vi "显示数据写入.vi"(0 "数组":u8[](array[numeric]), 5 "表格控件":string[][](table)) -> (4 "原始值1":string, 6 "实际值1":string, 8 "Function":string, 10 "address":string, 15 "所在表格行数":u16)   [LabVIEW 2018]
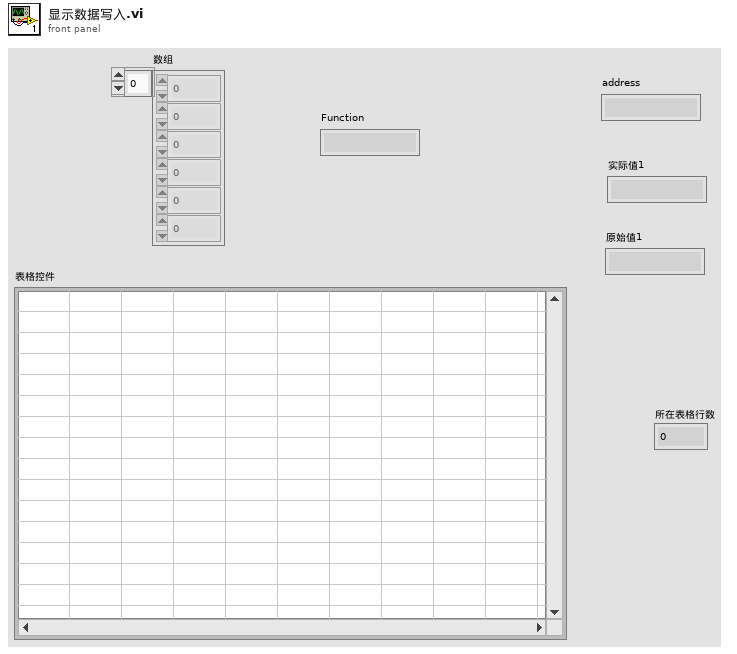
[diagram p1: front panel]
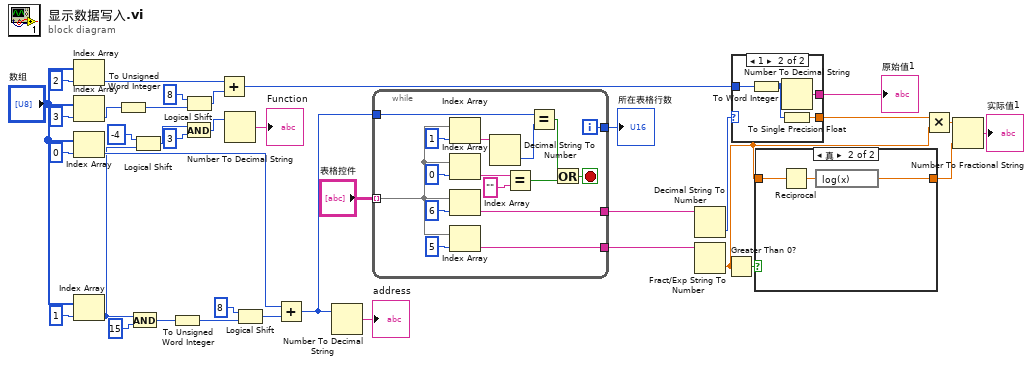
[diagram p0: block diagram]
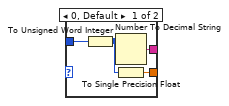
[diagram p2: hidden frame]
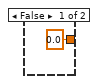
[diagram p3: hidden frame]
diagram:
  n1 = Index Array(array="数组", index=2 ("索引")) -> (element=w29:u8)
  n2 = Index Array(array="数组", index=3 ("索引")) -> (element=w2:u8)
  n3 = Index Array(array="数组", index=0 ("索引")) -> (element=w34:u8)
  n4 = Index Array(array="数组", index=1 ("索引")) -> (element=w7:u8)
  n5 = To Unsigned Word Integer(number=w2) -> (unsigned 16bit integer=w1:u16)
  n6 = And(x=w7, y=u8 15) -> (x .and. y?=w4:u8)
  n7 = Logical Shift(y=i16 -4, x=w7) -> (x << y=w5:u8)
  n8 = To Unsigned Word Integer(number=w4) -> (unsigned 16bit integer=w3:u16)
  n9 = Logical Shift(y=i16 8, x=w1) -> (x << y=w10:u16)
  n10 = And(x=w5, y=u16 3) -> (x .and. y?=w20:u16)
  n11 = Add(x=w29, y=w10) -> (x+y=w15:u16)
  n12 = Number To Decimal String(number=w20) -> (decimal integer string=→"Function":string)  [unwired: 1 in]
  n13 = Logical Shift(y=i16 8, x=w3) -> (x << y=w8:u16)
  n14 = Add(x=w34, y=w8) -> (x+y=w28:u16)
  n15 = Number To Decimal String(number=w28) -> (decimal integer string=→"address":string)  [unwired: 1 in]
  n16 = while {
    tunnel: "表格控件" -> [w40] mode=indexing
    tunnel: w28 -> [w50]
    tunnel: [w45] -> w27
    tunnel: [w41] -> w25
    tunnel: [w38] -> w16
    i -> [w41]
    stop <- w47 stop-if-true
    n17 = Index Array(array=w40, index=1 ("索引")) -> (element=w52:string)
    n18 = Index Array(array=w40, index=0 ("索引")) -> (element=w43:string)
    n19 = Index Array(array=w40, index=6 ("索引")) -> (element=w38:string)
    n20 = Index Array(array=w40, index=5 ("索引")) -> (element=w45:string)
    n21 = Decimal String To Number(string=w52) -> (number=w51:i32)  [unwired: 2 in, 1 out]
    n22 = Equal?(x=w43, y="") -> (x = y?=w48:bool)
    n23 = Equal?(x=w50, y=w51) -> (x = y?=w49:bool)
    n24 = Or(x=w49, y=w48) -> (x .or. y?=w47:bool)
  }
  "所在表格行数" <- w25
  n25 = Decimal String To Number(string=w16) -> (number=w13:i32)  [unwired: 2 in, 1 out]
  n26 = Fract/Exp String To Number(string=w27) -> (number=w18:dbl)  [unwired: 3 in, 1 out]
  n27 = Greater Than 0?(x=w18) -> (x > 0?=w23:bool)
  n28 = case shown="1" w13 {
    tunnel: w15 -> [w57 w61]
    tunnel: [w55 w59] -> w14
    tunnel: [w54 w58] -> w12
    frame 0, Default {
      n29 = To Unsigned Word Integer(number=w57) -> (unsigned 16bit integer=w56:u16)
      n30 = Number To Decimal String(number=w56) -> (decimal integer string=w54:string)  [unwired: 1 in]
      n31 = To Single Precision Float(number=w56) -> (single precision float=w55:sgl)
    }
    frame 1 {
      n32 = To Word Integer(number=w61) -> (16bit integer=w60:i16)
      n33 = Number To Decimal String(number=w60) -> (decimal integer string=w58:string)  [unwired: 1 in]
      n34 = To Single Precision Float(number=w60) -> (single precision float=w59:sgl)
    }
  }
  "原始值1" <- w12
  n35 = case shown="真" w23 {
    tunnel: w18 -> [_ w65]
    tunnel: [0.0 w63] -> w22
    frame False {
    }
    frame True {
      n36 = Reciprocal(x=w65) -> (1/x=w64:dbl)
      n37 = expression code="log(x)"(w64) -> (w63:dbl)
    }
  }
  n38 = Multiply(x=w14, y=w18) -> (x*y=w24:dbl)
  n39 = Number To Fractional String(number=w24, precision (6)=w22) -> (F-format string=→"实际值1":string)  [unwired: 2 in]
